vi "CalculateEmptyCaseStructureSizePosition.vi"(8 "error in (no error)":errorcluster, 11 "VI ref in":refnum<vi>) -> (0 "error out":errorcluster, 1 "Case structure frame size":T2, 2 "Case structure position":T1, 3 "VI ref (dup)":refnum<vi>)   [LabVIEW 2017, in "ErrorStructureDrawer.lvlib"]
doc: "Returns the size and position for drawing a case structure when there is nothing to put inside it. These values are based on the size of the visible block diagram, and on the developer configuration, which specifies the size of the empty case structure as a percentage of the visible block diagram.\n\nThe position is the top left external corner of the case structure when the structure is centered in the visible block diagram"
uses:
  ErrorStructureDrawer.lvlib
  <vilib>/Utility/miscctls.llb/LVBoundsTypeDef.ctl
  <vilib>/Utility/miscctls.llb/LVPositionTypeDef.ctl
  GetErrorStructureSize.vi
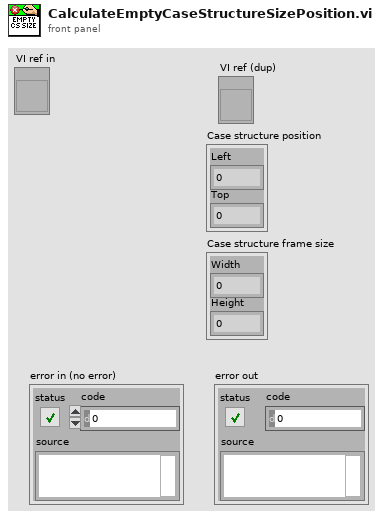
[diagram p1: front panel]
types:
  T1 = typedef "LVPositionTypeDef.ctl" = cluster{"Left":i32, "Top":i32}
  T2 = typedef "LVBoundsTypeDef.ctl" = cluster{"Width":u32, "Height":u32}
  T3 = typedef "LVPointTypeDef.ctl" = cluster{"Horizontal":i16, "Vertical":i16}
  T4 = typedef "ErrorStructureDrawer.lvlib/CaseStructureSizeIfBD_Empty.ctl" = cluster{"Width (%)":dbl, "Height (%)":dbl}
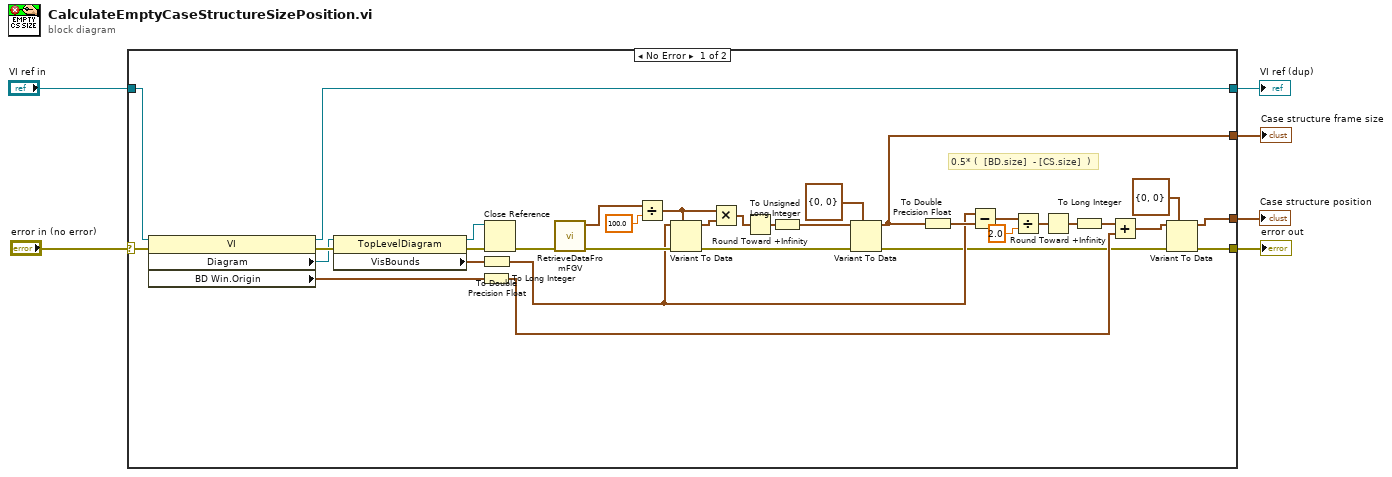
[diagram p0: block diagram]
diagram:
  n1 = case shown="No Error" "error in (no error)" {
    selector: "error in (no error)" -> [w18 w42]
    tunnel: [w9 _] -> w1
    tunnel: [w8 _] -> w6
    tunnel: [w11 w42] -> w5
    tunnel: "VI ref in" -> [w14 w41]
    tunnel: [w13 w41] -> w2
    frame No Error {
      # "0.5* (  [BD.size]  - [CS.size]  )"
      n2 = property class="VI"(reference=w14, error in=w18) -> (reference out=w13:refnum<vi>, error out=w24:errorcluster, "Diagram"=w23:refnum<vi>, "BD Win.Origin"=w21:T3)
      n3 = property class="TopLevelDiagram"(reference=w23, error in=w24) -> (reference out=w19:refnum<vi>, error out=w20:errorcluster, "VisBounds"=w22:T2)
      n4 = To Long Integer(number=w21) -> (32bit integer=w15:cluster{"Horizontal":i32, "Vertical":i32})
      n5 = To Double Precision Float(number=w22) -> (double precision float=w16:cluster{"Width":dbl, "Height":dbl})
      n6 = Close Reference(reference=w19, error in (no error)=w20) -> (error out=w17:errorcluster)
      n7 = call-poly "RetrieveDataFromFGV.vi"("error in (no error)"=w17) -> ("error out"=w37:errorcluster, "CS size if BD is empty"=w36:T4)  [unwired: 9 in]
      n8 = Divide(x=w36, y=100.0) -> (x/y=w39:T4)
      n9 = Variant To Data(error in=w37, type=w39, Variant=w16) -> (data=w38:T4, error out=w40:errorcluster)
      n10 = Multiply(x=w39, y=w38) -> (x*y=w25:T4)
      n11 = Round Toward +Infinity(x=w25) -> (ceil(x): smallest int >= x=w26:T4)
      n12 = To Unsigned Long Integer(number=w26) -> (unsigned 32bit integer=w30:cluster{"Width (%)":u32, "Height (%)":u32})
      n13 = Variant To Data(error in=w40, type=T2 {"Width"=0, "Height"=0} ("Bounding box for items in"), Variant=w30) -> (data=w8:T2, error out=w7:errorcluster)
      n14 = To Double Precision Float(number=w8) -> (double precision float=w32:cluster{"Width":dbl, "Height":dbl})
      n15 = Subtract(x=w16, y=w32) -> (x-y=w33:cluster{"Width":dbl, "Height":dbl})
      n16 = Divide(x=w33, y=2.0) -> (x/y=w35:cluster{"Width":dbl, "Height":dbl})
      n17 = Round Toward +Infinity(x=w35) -> (ceil(x): smallest int >= x=w34:cluster{"Width":dbl, "Height":dbl})
      n18 = To Long Integer(number=w34) -> (32bit integer=w31:cluster{"Width":i32, "Height":i32})
      n19 = Add(x=w31, y=w15) -> (x+y=w10:cluster{i32, i32})
      n20 = Variant To Data(error in=w7, type=T1 {"Left"=0, "Top"=0} ("position"), Variant=w10) -> (data=w9:T1, error out=w11:errorcluster)
    }
    frame Error {
    }
  }
  "error out" <- w5
  "Case structure frame size" <- w6
  "VI ref (dup)" <- w2
  "Case structure position" <- w1
